vi "SaveData Loop.vi"(8 "error in":errorcluster, 10 "Message Queues out":T14, 11 "Notifiers":T1) -> (0 "error out":errorcluster)   [LabVIEW 2014]
uses:
  support/Message Queue/All Message Queues.ctl
  support/Message Queue/Message Cluster.ctl
  support/Notifiers/Notifiers.ctl
  support/Message Handler Loop Notifiers.ctl
  Hardware Control/Parameter Analyzer/Parameter Analyzer Notifiers.ctl
  Hardware Control/Switching Matrix/Switching Matrix Notifiers.ctl
  Hardware Control/Stress Control/StressControl Notifiers.ctl
  Hardware Control/Spectrometer/Spectrometer Notifiers.ctl
  Hardware Control/Switches and Mirrors/SwitchesMirrors Notifiers.ctl
  Hardware Control/Camera/Camera Notifiers.ctl
  Hardware Control/XYZ Stage/XYZ Notifications.ctl
  Hardware Control/Autofocus/Autofocus Notifiers.ctl
  Measurements/Optoelectronic Measurement/Optoelectronic Notifiers.ctl
  Measurements/Save Data/SaveData Notifiers.ctl
  Measurements/Instrument Sequence/Instrument Sequence Notifiers.ctl
  Measurements/Save Data/SaveData Function.ctl
  support/Message Queue/Message Queue.lvlib
panel:
  # "LICENSED MATERIALS – PROPERTY OF IBM\nCopyright IBM Corp. 2016,\nALL RIGHTS RESERVED"
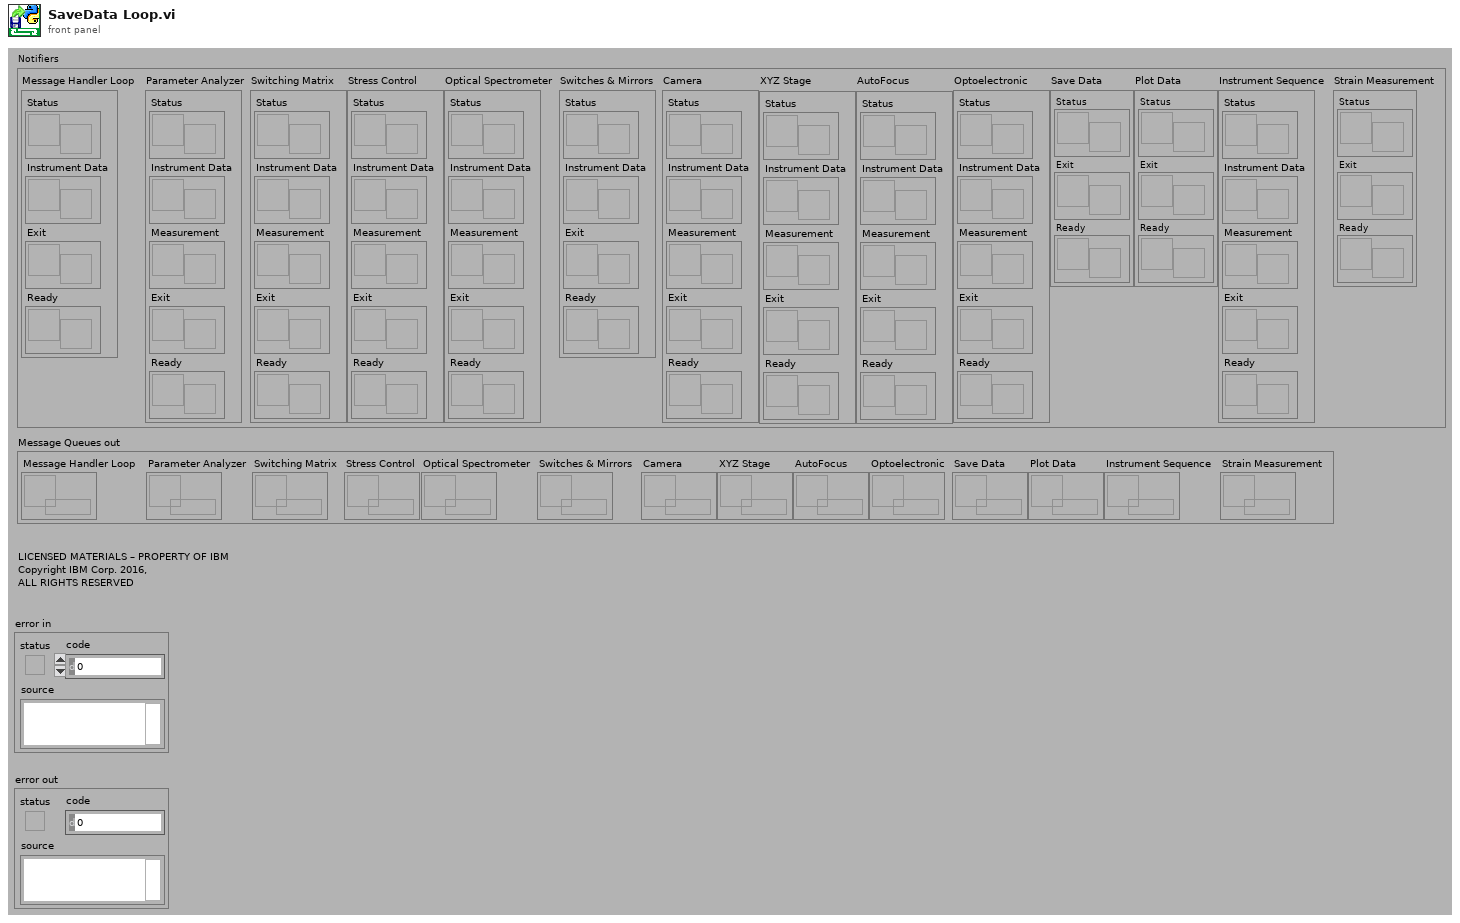
[diagram p1: front panel]
types:
  T1 = typedef "Notifiers.ctl" = cluster{"Message Handler Loop":T2, "Parameter Analyzer":T3, "Switching Matrix":T4, "Stress Control":T5, "Optical Spectrometer":T6, "Switches & Mirrors":T7, "Camera":T8, "XYZ Stage":T9, "AutoFocus":T10, "Optoelectronic":T11, "Save Data":T12, "Plot Data":T12, "Instrument Sequence":T13, "Strain Measurement":cluster{"Status":refnum<notifier>, "Exit":refnum<notifier>, "Ready":refnum<notifier>}}
  T2 = typedef "Message Handler Loop Notifiers.ctl" = cluster{"Status":refnum<notifier>, "Instrument Data":refnum<notifier>, "Exit":refnum<notifier>, "Ready":refnum<notifier>}
  T3 = typedef "Parameter Analyzer Notifiers.ctl" = cluster{"Status":refnum<notifier>, "Instrument Data":refnum<notifier>, "Measurement":refnum<notifier>, "Exit":refnum<notifier>, "Ready":refnum<notifier>}
  T4 = typedef "Switching Matrix Notifiers.ctl" = cluster{"Status":refnum<notifier>, "Instrument Data":refnum<notifier>, "Measurement":refnum<notifier>, "Exit":refnum<notifier>, "Ready":refnum<notifier>}
  T5 = typedef "StressControl Notifiers.ctl" = cluster{"Status":refnum<notifier>, "Instrument Data":refnum<notifier>, "Measurement":refnum<notifier>, "Exit":refnum<notifier>, "Ready":refnum<notifier>}
  T6 = typedef "Spectrometer Notifiers.ctl" = cluster{"Status":refnum<notifier>, "Instrument Data":refnum<notifier>, "Measurement":refnum<notifier>, "Exit":refnum<notifier>, "Ready":refnum<notifier>}
  T7 = typedef "SwitchesMirrors Notifiers.ctl" = cluster{"Status":refnum<notifier>, "Instrument Data":refnum<notifier>, "Exit":refnum<notifier>, "Ready":refnum<notifier>}
  T8 = typedef "Camera Notifiers.ctl" = cluster{"Status":refnum<notifier>, "Instrument Data":refnum<notifier>, "Measurement":refnum<notifier>, "Exit":refnum<notifier>, "Ready":refnum<notifier>}
  T9 = typedef "XYZ Notifications.ctl" = cluster{"Status":refnum<notifier>, "Instrument Data":refnum<notifier>, "Measurement":refnum<notifier>, "Exit":refnum<notifier>, "Ready":refnum<notifier>}
  T10 = typedef "Autofocus Notifiers.ctl" = cluster{"Status":refnum<notifier>, "Instrument Data":refnum<notifier>, "Measurement":refnum<notifier>, "Exit":refnum<notifier>, "Ready":refnum<notifier>}
  T11 = typedef "Optoelectronic Notifiers.ctl" = cluster{"Status":refnum<notifier>, "Instrument Data":refnum<notifier>, "Measurement":refnum<notifier>, "Exit":refnum<notifier>, "Ready":refnum<notifier>}
  T12 = typedef "SaveData Notifiers.ctl" = cluster{"Status":refnum<notifier>, "Exit":refnum<notifier>, "Ready":refnum<notifier>}
  T13 = typedef "Instrument Sequence Notifiers.ctl" = cluster{"Status":refnum<notifier>, "Instrument Data":refnum<notifier>, "Measurement":refnum<notifier>, "Exit":refnum<notifier>, "Ready":refnum<notifier>}
  T14 = typedef "Message Queue.lvlib/All Message Queues.ctl" = cluster{"Message Handler Loop":refnum<queue>, "Parameter Analyzer":refnum<queue>, "Switching Matrix":refnum<queue>, "Stress Control":refnum<queue>, "Optical Spectrometer":refnum<queue>, "Switches & Mirrors":refnum<queue>, "Camera":refnum<queue>, "XYZ Stage":refnum<queue>, "AutoFocus":refnum<queue>, "Optoelectronic":refnum<queue>, "Save Data":refnum<queue>, "Plot Data":refnum<queue>, "Instrument Sequence":refnum<queue>, "Strain Measurement":refnum<queue>}
  T15 = typedef "SaveData Function.ctl" = enum16{"Start Python Session", "Set Data Structures to Default", "Append Stress Data", "Append Electrical Measurement", "Append Optical Spectrum", "Append Stress Measurement Step", "Append Instrument Sequence Step", "Set Instrument Configuration", "Set Stress Data", "Set Electrical Measurement", "Set Optical Spectum", "Save Electrical Measurement", "Save Optical Spectrum", "Save Optoelectronic Measurement", "Save Instrument Sequence", "Save Stress Measurement", "Pickle2Workspace", "Explore Variable Space", "Close"}
  T16 = typedef "SaveData Data.ctl" = cluster{"Configuration":T17, "Initialization":T22}
  T17 = typedef "SaveData Config.ctl" = cluster{"Workspace Info":T18, "Instrument Configuration":T19, "Stress Motor Position":dbl, "Electrical Measurement":cluster{"Sequence":dbl[], "V1":dbl[], "V2":dbl[], "V3":dbl[], "V4":dbl[], "I1":dbl[], "I2":dbl[], "I3":dbl[], "I4":dbl[]}, "Optical Spectrum":T21}
  T18 = typedef "SaveData Workspace Info.ctl" = cluster{"Device Name":string, "Device Info":string, "Path":path}
  T19 = typedef "SaveData Instrument Configuration.ctl" = cluster{"Instrument":T20, "Configuration":string}
  T20 = typedef "Instrument List.ctl" = enum32{"Unknown Instrument", "Switching Matrix", "Parameter Analyzer", "Optical Spectrometer", "Optoelectronic", "Autofocus"}
  T21 = typedef "Spectral Data.ctl" = cluster{"Intensity":dbl[], "Wavelength":dbl[], "Energy":dbl[], "Raman Shift":dbl[], "Detector Temperature":dbl}
  T22 = typedef "SaveData Initialization.ctl" = cluster{"Start Python Session":bool, "Set Datastructures to Default":bool}
  T23 = cluster{"Sequence":dbl[], "V1":dbl[], "V2":dbl[], "V3":dbl[], "V4":dbl[], "I1":dbl[], "I2":dbl[], "I3":dbl[], "I4":dbl[]}
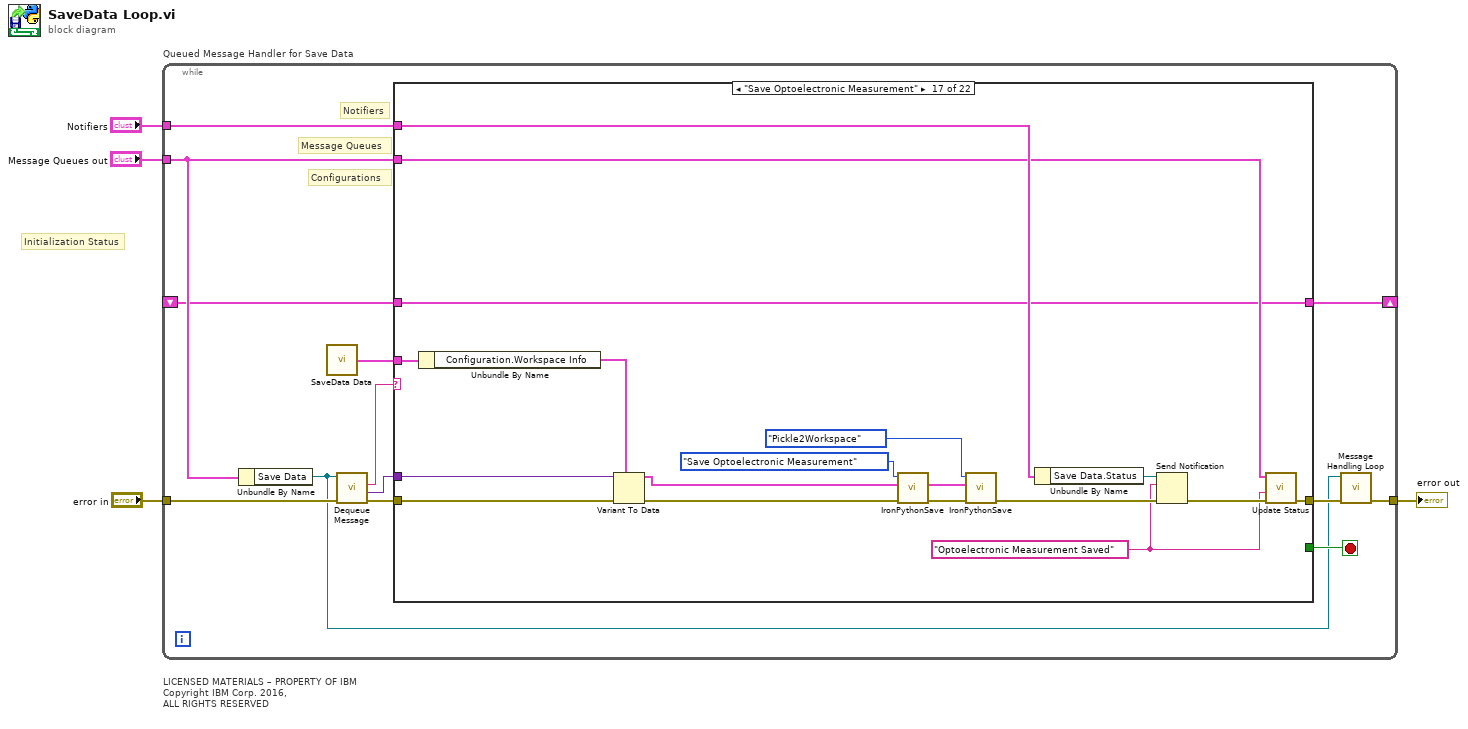
[diagram p0: block diagram]
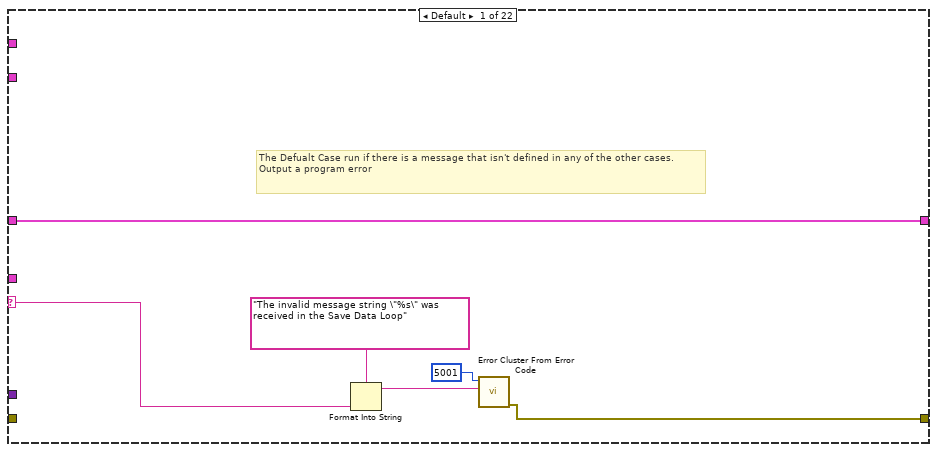
[diagram p2: hidden frame]
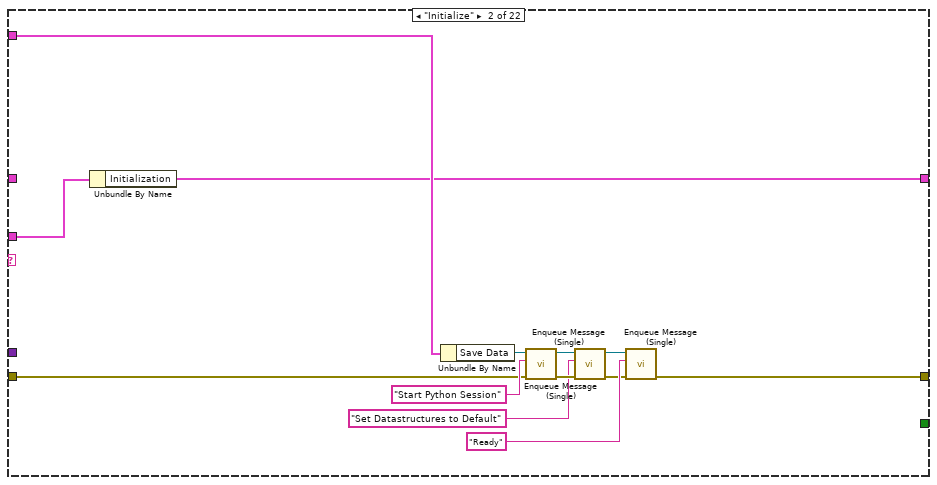
[diagram p3: hidden frame]
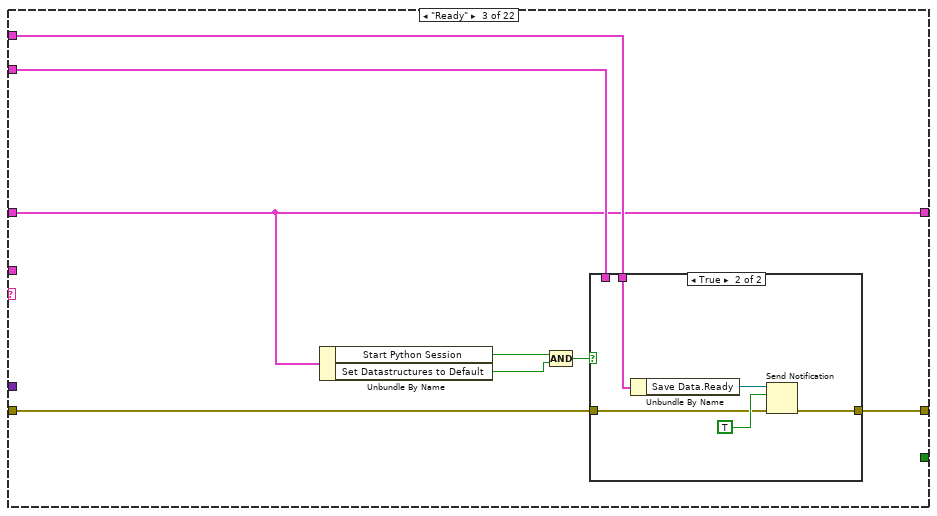
[diagram p4: hidden frame]
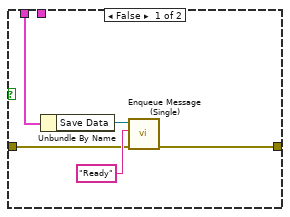
[diagram p5: hidden frame]
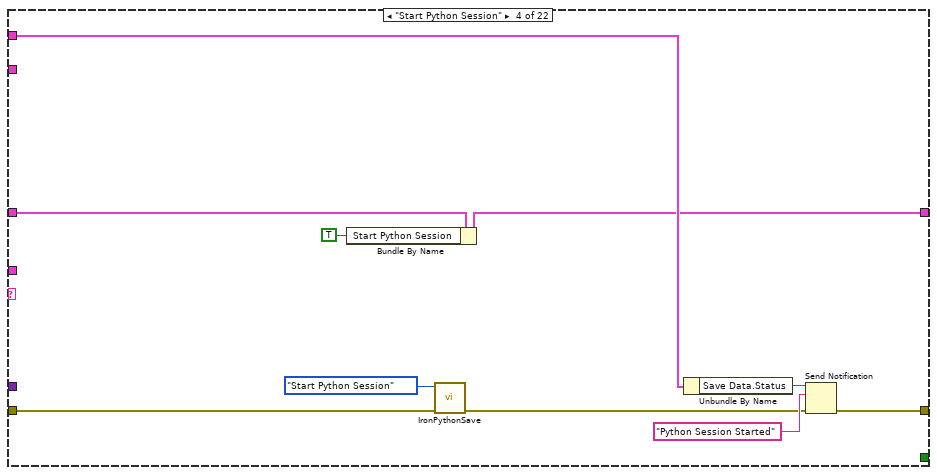
[diagram p6: hidden frame]
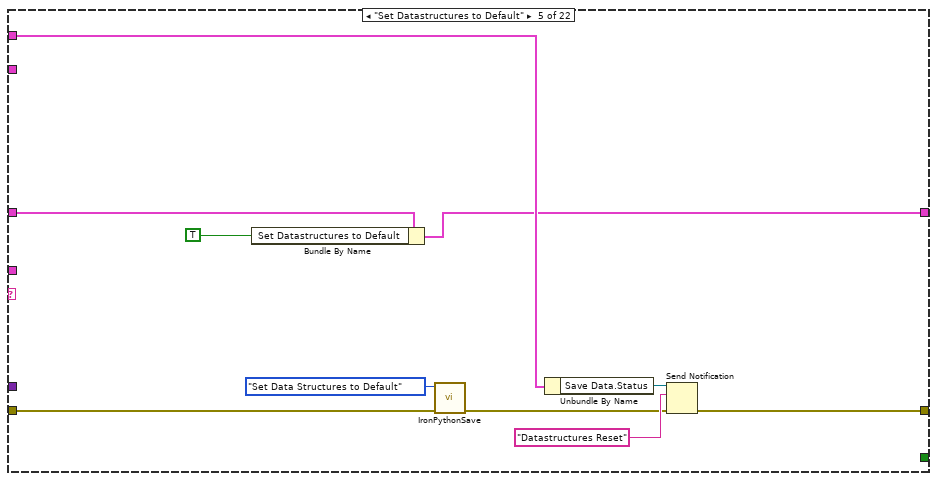
[diagram p7: hidden frame]
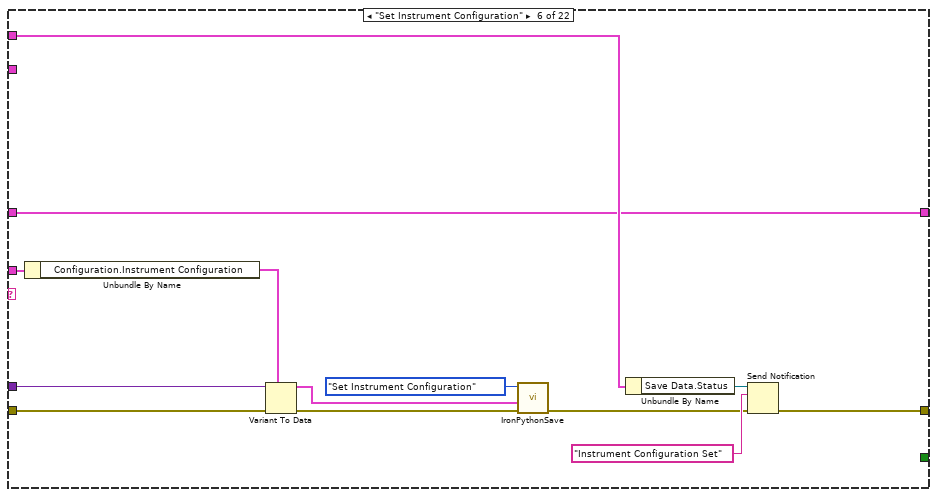
[diagram p8: hidden frame]
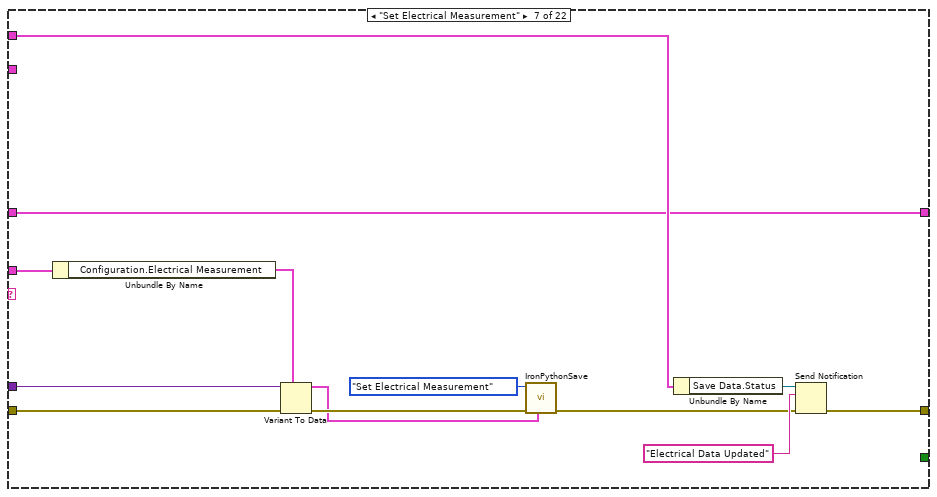
[diagram p9: hidden frame]
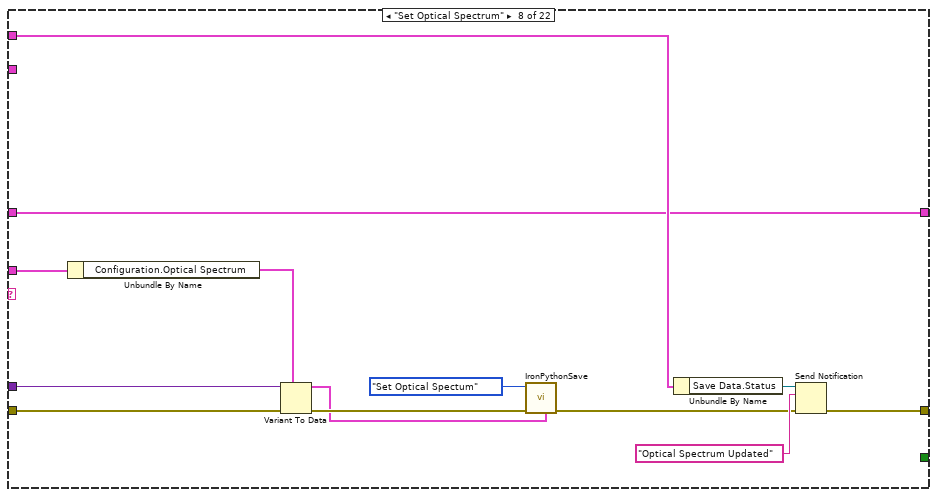
[diagram p10: hidden frame]
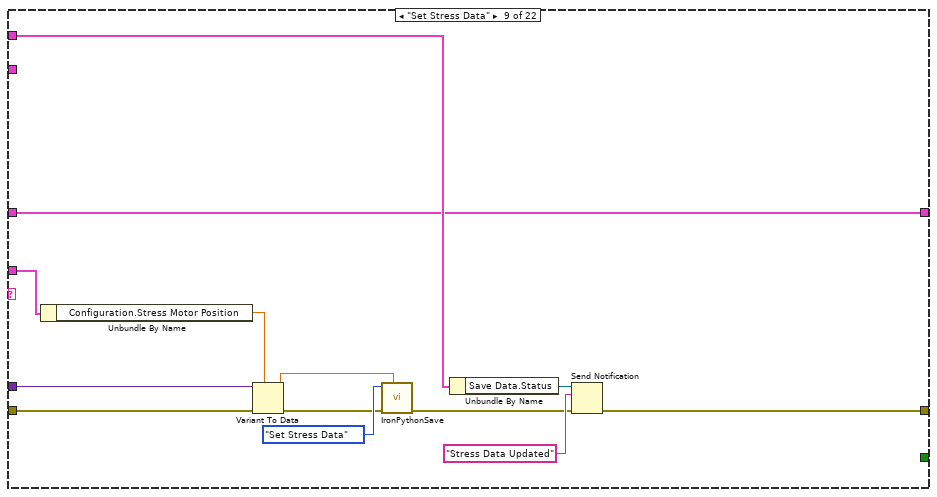
[diagram p11: hidden frame]
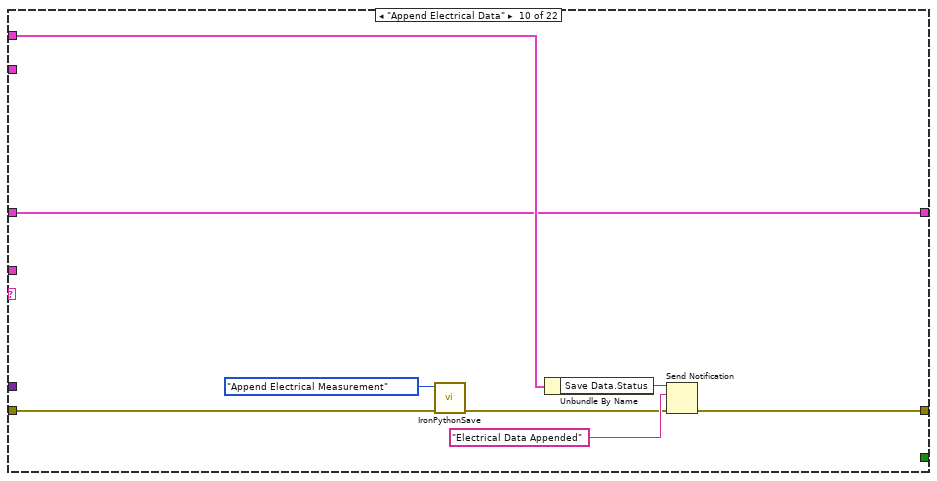
[diagram p12: hidden frame]
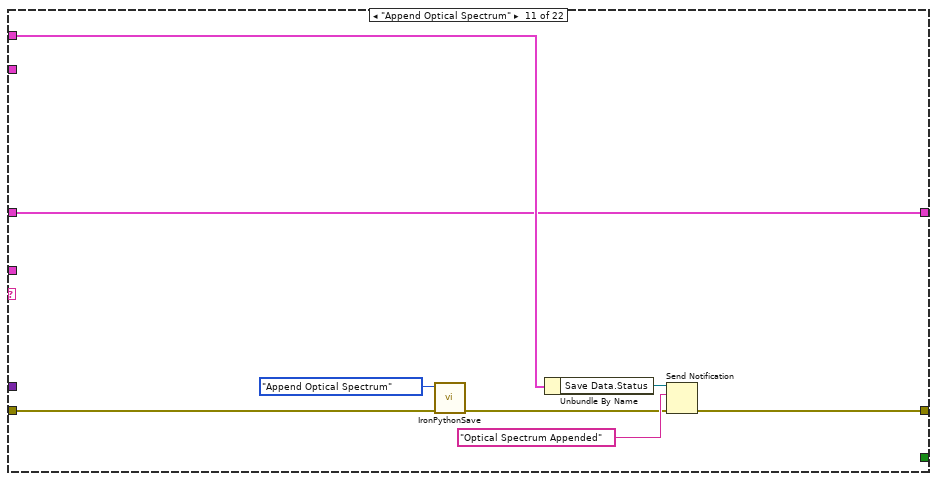
[diagram p13: hidden frame]
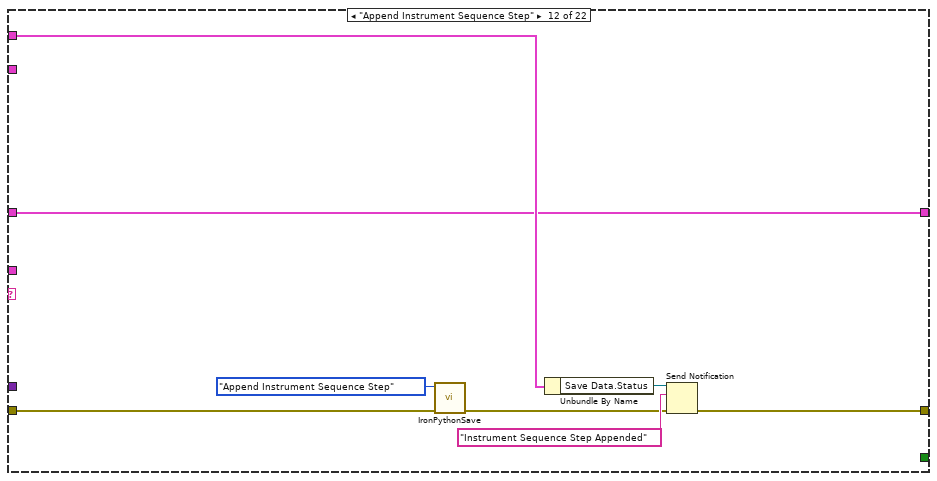
[diagram p14: hidden frame]
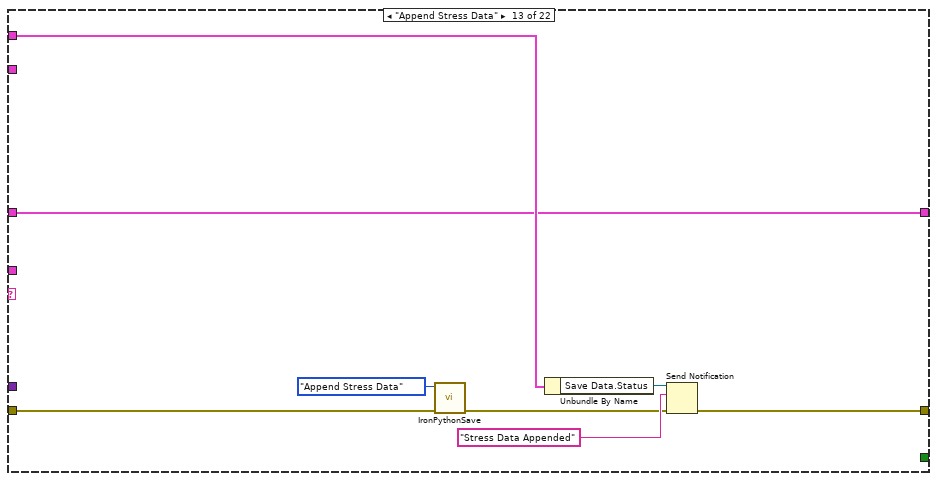
[diagram p15: hidden frame]
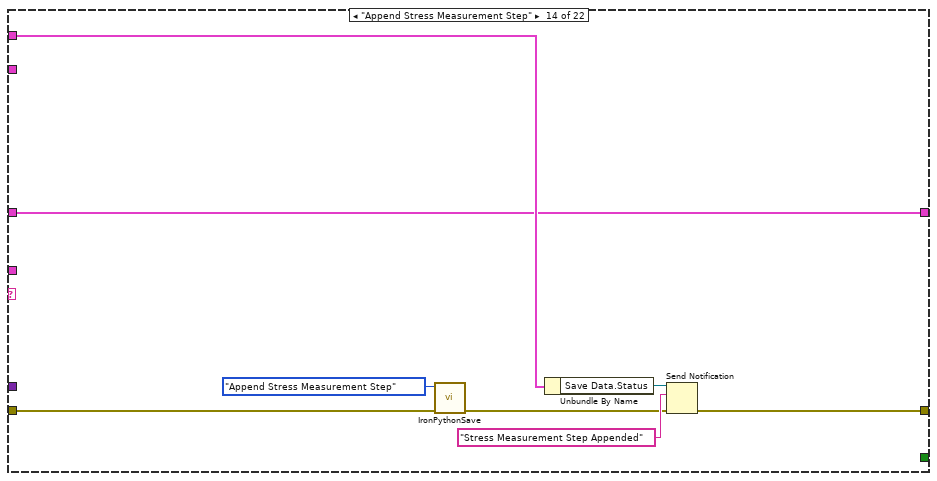
[diagram p16: hidden frame]
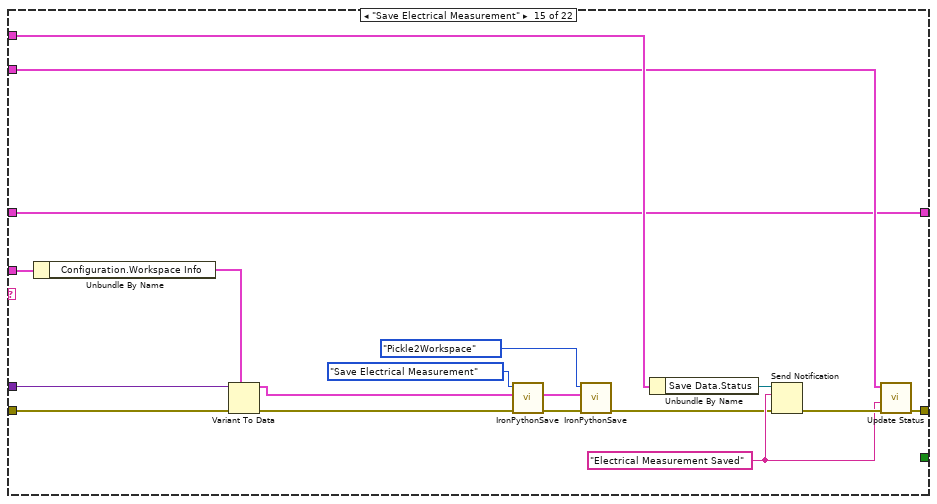
[diagram p17: hidden frame]
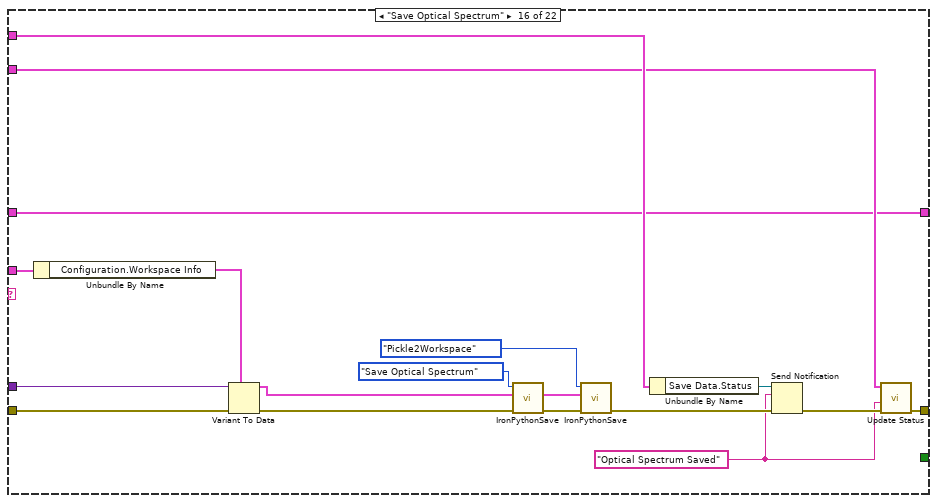
[diagram p18: hidden frame]
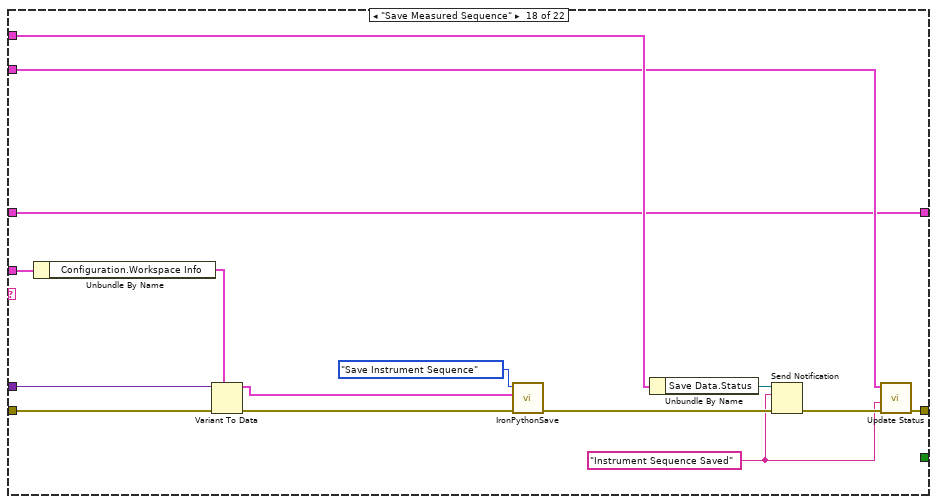
[diagram p19: hidden frame]
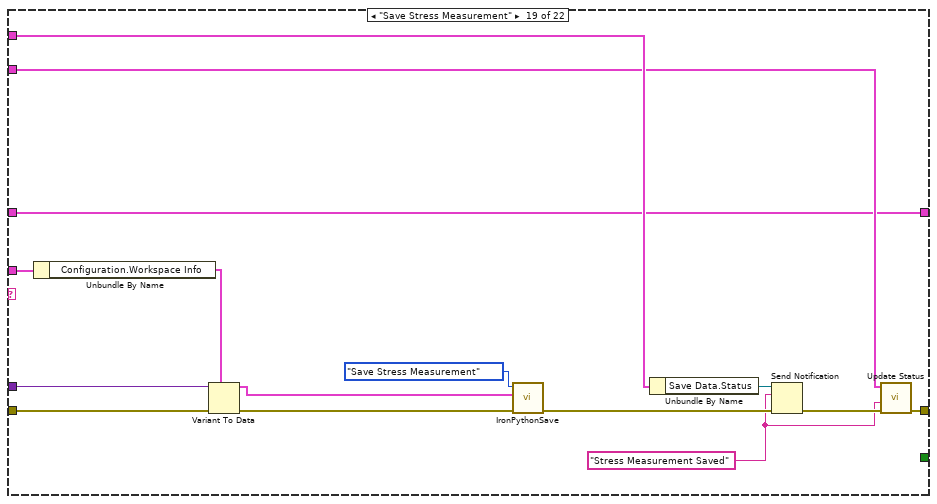
[diagram p20: hidden frame]
diagram:
  # "LICENSED MATERIALS – PROPERTY OF IBM\nCopyright IBM Corp. 2016,\nALL RIGHTS RESERVED"
  # "Initialization Status"
  n1 = while "Queued Message Handler for Save Data" {
    tunnel: "error in" -> [w17]
    tunnel: [w9] -> w1
    tunnel: "Message Queues out" -> [w13]
    tunnel: "Notifiers" -> [w12]
    shift-right: [w6] -> _
    shift-left: _ -> [w5]
    stop <- w11 stop-if-true
    # "Configurations"
    # "Notifiers"
    # "Message Queues"
    n2 = Unbundle By Name(w13) -> ("Save Data"=w8:refnum<queue>)
    n3 = call "SaveData Data.vi"() -> ("SavaData Data"=w7:T16)
    n4 = call "Dequeue Message.vi"("error in (no error)"=w17, "Message Queue"=w8) -> ("error out"=w16:errorcluster, "Message Data"=w14:variant, "Message"=w15:string)  [unwired: 7 out]
    n5 = case shown="\"Save Optoelectronic Measurement\"" w15 {
      selector: w15 -> [w20 _ _ _ _ _ _ _ _ _ _ _ _ _ _ _ _ _ _ _ _ _]
      tunnel: w16 -> [_ w33 w44 w62 w72 w87 w100 w113 w126 w133 w141 w149 w157 w165 w183 w200 w217 w232 w247 w264 w273 w291]
      tunnel: [w19 w26 w42 w57 w67 w78 w90 w104 w116 w128 w136 w144 w152 w160 w178 w195 w212 w227 w242 w259 w268 w281] -> w10
      tunnel: w14 -> [_ _ _ _ _ w86 w99 w112 w125 _ _ _ _ _ w182 w199 w216 w231 w246 w263 w266 _]
      tunnel: w13 -> [_ w36 w43 _ _ _ _ _ _ _ _ _ _ _ w179 w196 w213 w228 w243 w260 w274 w293]
      tunnel: w12 -> [_ _ w41 w59 w69 w85 w98 w111 w124 w130 w138 w146 w154 w162 w181 w198 w215 w230 w245 w262 _ w283]
      tunnel: [_ _ _ _ _ _ _ _ _ _ _ _ _ _ _ _ _ _ _ _ _ TRUE ("Priority Message? (F)")] -> w11
      tunnel: w7 -> [_ w25 _ _ _ w77 w89 w103 w115 _ _ _ _ _ w172 w190 w207 w220 w235 w253 _ _]
      tunnel: [w18 w24 w37 w56 w65 w75 w88 w102 w114 w127 w135 w143 w151 w159 w171 w189 w206 w219 w234 w252 w265 w288] -> w6
      tunnel: w5 -> [w18 _ w37 w55 w66 w75 w88 w102 w114 w127 w135 w143 w151 w159 w171 w189 w206 w219 w234 w252 w265 w288]
      frame Default {
        # "The Defualt Case run if there is a message that isn't defined in any of the other cases.\nOutput a program error"
        n6 = Format Into String(format string="The invalid message string \"%s\" was  received in the Save Data Loop", w20) -> (resulting string=w22:string)  [unwired: 2 in, 1 out]
        n7 = call <vilib>:"Error Cluster From Error Code.vi"("error message (\"\")"=w22, "error code (0)"=5001) -> ("error out"=w19:errorcluster)  [unwired: 2 in, 5 out]
      }
      frame "Initialize" {
        n8 = Unbundle By Name(w25) -> ("Initialization"=w24:T22)
        n9 = Unbundle By Name(w36) -> ("Save Data"=w34:refnum<queue>)
        n10 = call "Enqueue Message (Single).vi"("error in (no error)"=w33, "Message"="Start Python Session", "Message Queue"=w34) -> ("error out"=w32:errorcluster, "dup Message Queue"=w31:refnum<queue>)  [unwired: 1 in, 6 out]
        n11 = call "Enqueue Message (Single).vi"("error in (no error)"=w32, "Message"="Set Datastructures to Default", "Message Queue"=w31) -> ("error out"=w27:errorcluster, "dup Message Queue"=w29:refnum<queue>)  [unwired: 1 in, 6 out]
        n12 = call "Enqueue Message (Single).vi"("error in (no error)"=w27, "Message"="Ready", "Message Queue"=w29) -> ("error out"=w26:errorcluster)  [unwired: 1 in, 7 out]
      }
      frame "Ready" {
        n13 = Unbundle By Name(w37) -> ("Start Python Session"=w40:bool, "Set Datastructures to Default"=w38:bool)
        n14 = Compound Arithmetic op=AND(w40, w38) -> (w39:bool)
        n15 = case shown="True" w39 {
          tunnel: [w47 w52] -> w42
          tunnel: w44 -> [w46 w51]
          tunnel: w43 -> [w45 _]
          tunnel: w41 -> [_ w50]
          frame False {
            n16 = Unbundle By Name(w45) -> ("Save Data"=w49:refnum<queue>)
            n17 = call "Enqueue Message (Single).vi"("error in (no error)"=w46, "Message"="Ready", "Message Queue"=w49) -> ("error out"=w47:errorcluster)  [unwired: 1 in, 7 out]
          }
          frame True {
            n18 = Unbundle By Name(w50) -> ("Save Data.Ready"=w53:refnum<notifier>)
            n19 = Send Notification(notification=TRUE, notifier=w53, error in (no error)=w51) -> (error out=w52:errorcluster)  [unwired: 1 out]
          }
        }
      }
      frame "Start Python Session" {
        n20 = Bundle By Name(cluster=w55, "Start Python Session"=TRUE ("Initialization.Open VI reference")) -> (w56:T22)
        n21 = call "IronPythonSave.vi"("error in (no error)"=w62, "Function"=SaveData_Function."Start Python Session") -> ("error out"=w58:errorcluster)  [unwired: 9 in]
        n22 = Unbundle By Name(w59) -> ("Save Data.Status"=w60:refnum<notifier>)
        n23 = Send Notification(notification="Python Session Started", notifier=w60, error in (no error)=w58) -> (error out=w57:errorcluster)  [unwired: 1 out]
      }
      frame "Set Datastructures to Default" {
        n24 = Bundle By Name(cluster=w66, "Set Datastructures to Default"=TRUE ("Initialization.Open VI reference")) -> (w65:T22)
        n25 = call "IronPythonSave.vi"("error in (no error)"=w72, "Function"=SaveData_Function."Set Data Structures to Default") -> ("error out"=w68:errorcluster)  [unwired: 9 in]
        n26 = Unbundle By Name(w69) -> ("Save Data.Status"=w70:refnum<notifier>)
        n27 = Send Notification(notification="Datastructures Reset", notifier=w70, error in (no error)=w68) -> (error out=w67:errorcluster)  [unwired: 1 out]
      }
      frame "Set Instrument Configuration" {
        n28 = Unbundle By Name(w77) -> ("Configuration.Instrument Configuration"=w84:T19)
        n29 = Variant To Data(error in=w87, type=w84, Variant=w86) -> (data=w76:T19, error out=w79:errorcluster)
        n30 = call "IronPythonSave.vi"("error in (no error)"=w79, "Instrument Configuration"=w76, "Function"=SaveData_Function."Set Instrument Configuration") -> ("error out"=w80:errorcluster)  [unwired: 8 in]
        n31 = Unbundle By Name(w85) -> ("Save Data.Status"=w82:refnum<notifier>)
        n32 = Send Notification(notification="Instrument Configuration Set", notifier=w82, error in (no error)=w80) -> (error out=w78:errorcluster)  [unwired: 1 out]
      }
      frame "Set Electrical Measurement" {
        n33 = Unbundle By Name(w89) -> ("Configuration.Electrical Measurement"=w97:T23)
        n34 = Variant To Data(error in=w100, type=w97, Variant=w99) -> (data=w91:T23, error out=w92:errorcluster)
        n35 = call "IronPythonSave.vi"("Electrical Measurement"=w91, "error in (no error)"=w92, "Function"=SaveData_Function."Set Electrical Measurement") -> ("error out"=w93:errorcluster)  [unwired: 8 in]
        n36 = Unbundle By Name(w98) -> ("Save Data.Status"=w95:refnum<notifier>)
        n37 = Send Notification(notification="Electrical Data Updated", notifier=w95, error in (no error)=w93) -> (error out=w90:errorcluster)  [unwired: 1 out]
      }
      frame "Set Optical Spectrum" {
        n38 = Unbundle By Name(w103) -> ("Configuration.Optical Spectrum"=w110:T21)
        n39 = Variant To Data(error in=w113, type=w110, Variant=w112) -> (data=w101:T21, error out=w105:errorcluster)
        n40 = call "IronPythonSave.vi"("Optical Spectrum"=w101, "error in (no error)"=w105, "Function"=SaveData_Function."Set Optical Spectum") -> ("error out"=w106:errorcluster)  [unwired: 8 in]
        n41 = Unbundle By Name(w111) -> ("Save Data.Status"=w108:refnum<notifier>)
        n42 = Send Notification(notification="Optical Spectrum Updated", notifier=w108, error in (no error)=w106) -> (error out=w104:errorcluster)  [unwired: 1 out]
      }
      frame "Set Stress Data" {
        n43 = Unbundle By Name(w115) -> ("Configuration.Stress Motor Position"=w123:dbl)
        n44 = Variant To Data(error in=w126, type=w123, Variant=w125) -> (data=w117:dbl, error out=w118:errorcluster)
        n45 = call "IronPythonSave.vi"("Stress Motor Position"=w117, "error in (no error)"=w118, "Function"=SaveData_Function."Set Stress Data") -> ("error out"=w119:errorcluster)  [unwired: 8 in]
        n46 = Unbundle By Name(w124) -> ("Save Data.Status"=w121:refnum<notifier>)
        n47 = Send Notification(notification="Stress Data Updated", notifier=w121, error in (no error)=w119) -> (error out=w116:errorcluster)  [unwired: 1 out]
      }
      frame "Append Electrical Data" {
        n48 = call "IronPythonSave.vi"("error in (no error)"=w133, "Function"=SaveData_Function."Append Electrical Measurement") -> ("error out"=w129:errorcluster)  [unwired: 9 in]
        n49 = Unbundle By Name(w130) -> ("Save Data.Status"=w131:refnum<notifier>)
        n50 = Send Notification(notification="Electrical Data Appended", notifier=w131, error in (no error)=w129) -> (error out=w128:errorcluster)  [unwired: 1 out]
      }
      frame "Append Optical Spectrum" {
        n51 = call "IronPythonSave.vi"("error in (no error)"=w141, "Function"=SaveData_Function."Append Optical Spectrum") -> ("error out"=w137:errorcluster)  [unwired: 9 in]
        n52 = Unbundle By Name(w138) -> ("Save Data.Status"=w139:refnum<notifier>)
        n53 = Send Notification(notification="Optical Spectrum Appended", notifier=w139, error in (no error)=w137) -> (error out=w136:errorcluster)  [unwired: 1 out]
      }
      frame "Append Instrument Sequence Step" {
        n54 = call "IronPythonSave.vi"("error in (no error)"=w149, "Function"=SaveData_Function."Append Instrument Sequence Step") -> ("error out"=w145:errorcluster)  [unwired: 9 in]
        n55 = Unbundle By Name(w146) -> ("Save Data.Status"=w147:refnum<notifier>)
        n56 = Send Notification(notification="Instrument Sequence Step Appended", notifier=w147, error in (no error)=w145) -> (error out=w144:errorcluster)  [unwired: 1 out]
      }
      frame "Append Stress Data" {
        n57 = call "IronPythonSave.vi"("error in (no error)"=w157, "Function"=SaveData_Function."Append Stress Data") -> ("error out"=w153:errorcluster)  [unwired: 9 in]
        n58 = Unbundle By Name(w154) -> ("Save Data.Status"=w155:refnum<notifier>)
        n59 = Send Notification(notification="Stress Data Appended", notifier=w155, error in (no error)=w153) -> (error out=w152:errorcluster)  [unwired: 1 out]
      }
      frame "Append Stress Measurement Step" {
        n60 = call "IronPythonSave.vi"("error in (no error)"=w165, "Function"=SaveData_Function."Append Stress Measurement Step") -> ("error out"=w161:errorcluster)  [unwired: 9 in]
        n61 = Unbundle By Name(w162) -> ("Save Data.Status"=w163:refnum<notifier>)
        n62 = Send Notification(notification="Stress Measurement Step Appended", notifier=w163, error in (no error)=w161) -> (error out=w160:errorcluster)  [unwired: 1 out]
      }
      frame "Save Electrical Measurement" {
        w173 = "Electrical Measurement Saved"
        n63 = Unbundle By Name(w172) -> ("Configuration.Workspace Info"=w176:T18)
        n64 = Variant To Data(error in=w183, type=w176, Variant=w182) -> (data=w167:T18, error out=w174:errorcluster)
        n65 = call "IronPythonSave.vi"("error in (no error)"=w174, "Workspace Info"=w167, "Function"=SaveData_Function."Save Electrical Measurement") -> ("error out"=w169:errorcluster)  [unwired: 8 in]
        n66 = call "IronPythonSave.vi"("error in (no error)"=w169, "Workspace Info"=w167, "Function"=SaveData_Function."Pickle2Workspace") -> ("error out"=w168:errorcluster)  [unwired: 8 in]
        n67 = Unbundle By Name(w181) -> ("Save Data.Status"=w177:refnum<notifier>)
        n68 = Send Notification(notification=w173, notifier=w177, error in (no error)=w168) -> (error out=w180:errorcluster)  [unwired: 1 out]
        n69 = call "Update Status.vi"("error in"=w180, "String"=w173, "Message Queues out"=w179) -> ("error out"=w178:errorcluster)  [unwired: 8 out]
      }
      frame "Save Optical Spectrum" {
        w184 = "Optical Spectrum Saved"
        n70 = Unbundle By Name(w190) -> ("Configuration.Workspace Info"=w193:T18)
        n71 = Variant To Data(error in=w200, type=w193, Variant=w199) -> (data=w185:T18, error out=w191:errorcluster)
        n72 = call "IronPythonSave.vi"("error in (no error)"=w191, "Workspace Info"=w185, "Function"=SaveData_Function."Save Optical Spectrum") -> ("error out"=w187:errorcluster)  [unwired: 8 in]
        n73 = call "IronPythonSave.vi"("error in (no error)"=w187, "Workspace Info"=w185, "Function"=SaveData_Function."Pickle2Workspace") -> ("error out"=w186:errorcluster)  [unwired: 8 in]
        n74 = Unbundle By Name(w198) -> ("Save Data.Status"=w194:refnum<notifier>)
        n75 = Send Notification(notification=w184, notifier=w194, error in (no error)=w186) -> (error out=w197:errorcluster)  [unwired: 1 out]
        n76 = call "Update Status.vi"("error in"=w197, "String"=w184, "Message Queues out"=w196) -> ("error out"=w195:errorcluster)  [unwired: 8 out]
      }
      frame "Save Optoelectronic Measurement" {
        w201 = "Optoelectronic Measurement Saved"
        n77 = Unbundle By Name(w207) -> ("Configuration.Workspace Info"=w210:T18)
        n78 = Variant To Data(error in=w217, type=w210, Variant=w216) -> (data=w202:T18, error out=w208:errorcluster)
        n79 = call "IronPythonSave.vi"("error in (no error)"=w208, "Workspace Info"=w202, "Function"=SaveData_Function."Save Optoelectronic Measurement") -> ("error out"=w204:errorcluster)  [unwired: 8 in]
        n80 = call "IronPythonSave.vi"("error in (no error)"=w204, "Workspace Info"=w202, "Function"=SaveData_Function."Pickle2Workspace") -> ("error out"=w203:errorcluster)  [unwired: 8 in]
        n81 = Unbundle By Name(w215) -> ("Save Data.Status"=w211:refnum<notifier>)
        n82 = Send Notification(notification=w201, notifier=w211, error in (no error)=w203) -> (error out=w214:errorcluster)  [unwired: 1 out]
        n83 = call "Update Status.vi"("error in"=w214, "String"=w201, "Message Queues out"=w213) -> ("error out"=w212:errorcluster)  [unwired: 8 out]
      }
      frame "Save Measured Sequence" {
        w221 = "Instrument Sequence Saved"
        n84 = Unbundle By Name(w220) -> ("Configuration.Workspace Info"=w225:T18)
        n85 = Variant To Data(error in=w232, type=w225, Variant=w231) -> (data=w218:T18, error out=w222:errorcluster)
        n86 = call "IronPythonSave.vi"("error in (no error)"=w222, "Workspace Info"=w218, "Function"=SaveData_Function."Save Instrument Sequence") -> ("error out"=w223:errorcluster)  [unwired: 8 in]
        n87 = Unbundle By Name(w230) -> ("Save Data.Status"=w226:refnum<notifier>)
        n88 = Send Notification(notification=w221, notifier=w226, error in (no error)=w223) -> (error out=w229:errorcluster)  [unwired: 1 out]
        n89 = call "Update Status.vi"("error in"=w229, "String"=w221, "Message Queues out"=w228) -> ("error out"=w227:errorcluster)  [unwired: 8 out]
      }
      frame "Save Stress Measurement" {
        w236 = "Stress Measurement Saved"
        n90 = Unbundle By Name(w235) -> ("Configuration.Workspace Info"=w240:T18)
        n91 = Variant To Data(error in=w247, type=w240, Variant=w246) -> (data=w233:T18, error out=w237:errorcluster)
        n92 = call "IronPythonSave.vi"("error in (no error)"=w237, "Workspace Info"=w233, "Function"=SaveData_Function."Save Stress Measurement") -> ("error out"=w238:errorcluster)  [unwired: 8 in]
        n93 = Unbundle By Name(w245) -> ("Save Data.Status"=w241:refnum<notifier>)
        n94 = Send Notification(notification=w236, notifier=w241, error in (no error)=w238) -> (error out=w244:errorcluster)  [unwired: 1 out]
        n95 = call "Update Status.vi"("error in"=w244, "String"=w236, "Message Queues out"=w243) -> ("error out"=w242:errorcluster)  [unwired: 8 out]
      }
      frame "Pickle2Workspace" {
        w254 = "Workspace file saved"
        n96 = Unbundle By Name(w253) -> ("Configuration.Workspace Info"=w257:T18)
        n97 = Variant To Data(error in=w264, type=w257, Variant=w263) -> (data=w248:T18, error out=w255:errorcluster)
        n98 = call "IronPythonSave.vi"("error in (no error)"=w255, "Workspace Info"=w248, "Function"=SaveData_Function."Pickle2Workspace") -> ("error out"=w250:errorcluster)  [unwired: 8 in]
        n99 = call "IronPythonSave.vi"("error in (no error)"=w250, "Function"=SaveData_Function."Set Data Structures to Default") -> ("error out"=w249:errorcluster)  [unwired: 9 in]
        n100 = Unbundle By Name(w262) -> ("Save Data.Status"=w258:refnum<notifier>)
        n101 = Send Notification(notification=w254, notifier=w258, error in (no error)=w249) -> (error out=w261:errorcluster)  [unwired: 1 out]
        n102 = call "Update Status.vi"("error in"=w261, "String"=w254, "Message Queues out"=w260) -> ("error out"=w259:errorcluster)  [unwired: 8 out]
      }
      frame "Error" {
        # "Clear Errors to avoid getting stuck \nin repeating this case"
        # "Add here Cases that are handled \nalready by the Message Handler Loop"
        n103 = Variant To Data(error in=w273, type=errorcluster {"status"=FALSE, "code"=0, "source"=""} ("error out"), Variant=w266) -> (data=w272:errorcluster, error out=w271:errorcluster)
        n104 = Merge Errors(w272, w271) -> (w270:errorcluster)
        n105 = Unbundle By Name(w274) -> ("Message Handler Loop"=w276:refnum<queue>)
        n106 = Unbundle By Name(w270) -> ("code"=w267:i32)
        n107 = case shown="Default" w267 {
          tunnel: w276 -> [w280]
          tunnel: w270 -> [w278]
          tunnel: [w277] -> w269
          frame Default {
            n108 = call "Enqueue Message (Single).vi"("Message Data"=w278, "Message"="Error", "Message Queue"=w280) -> ("error out"=w277:errorcluster)  [unwired: 1 in, 7 out]
          }
        }
        n109 = call <vilib>:"Clear Errors.vi"("error in (no error)"=w269) -> ("error out"=w268:errorcluster)  [unwired: 1 in, 5 out]
      }
      frame "Exit" {
        w286 = TRUE ("Priority Message? (F)")
        # "Stop the VI"
        n110 = call "IronPythonSave.vi"("error in (no error)"=w291, "Function"=SaveData_Function."Close") -> ("error out"=w290:errorcluster)  [unwired: 9 in]
        n111 = Unbundle By Name(w293) -> ("Save Data"=w294:refnum<queue>)
        n112 = Release Queue(queue=w294, error in (no error)=w290) -> (error out=w282:errorcluster)  [unwired: 3 out]
        n113 = Unbundle By Name(w283) -> ("Save Data.Exit"=w287:refnum<notifier>, "Save Data.Ready"=w284:refnum<notifier>)
        n114 = Send Notification(notification=w286, notifier=w284, error in (no error)=w282) -> (error out=w285:errorcluster)  [unwired: 1 out]
        n115 = Send Notification(notification=w286, notifier=w287, error in (no error)=w285) -> (error out=w281:errorcluster)  [unwired: 1 out]
      }
    }
    n116 = call "Message Handling Loop.vi"("error in (no error)"=w10, "Message Queue"=w8) -> ("dup error in"=w9:errorcluster)  [unwired: 9 out]
  }
  "error out" <- w1
